vi "Close RF Subsystem Sessions.vi"(0 "RF SubSystem Session Providers":refnum<class "RF Subsystem Session Provider.lvclass">[](array[class]), 5 "TSM Context":T1, 11 "Error in":errorcluster) -> (15 "Error out":errorcluster)   [LabVIEW 2023, in "RFCalAndFixtureCharact.Common.lvlib"]
uses:
  RFCalAndFixtureCharact.Common.lvlib
  <vilib>/NI_TestStand_SemiconductorModule/NI_TestStand_Semiconductor_Module.lvlibp/PinMap/General/SemiconductorModuleContext.ctl
  RF Subsystem Session Provider/RF Subsystem Session Provider.lvclass
  <vilib>/NI_TestStand_SemiconductorModule/NI_TestStand_Semiconductor_Module.lvlibp
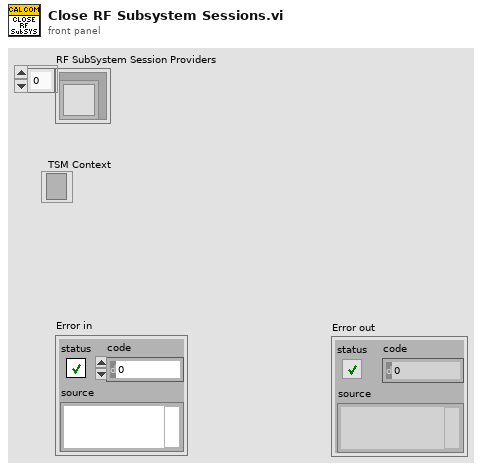
[diagram p1: front panel]
types:
  T1 = typedef "NI_TestStand_Semiconductor_Module.lvlibp/SemiconductorModuleContext.ctl" = refnum<k7>
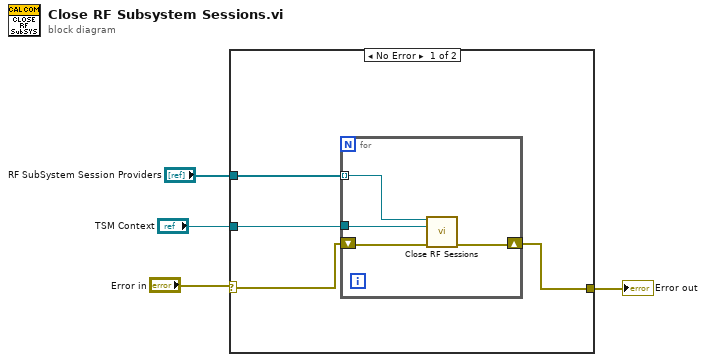
[diagram p0: block diagram]
diagram:
  n1 = case shown="No Error" "Error in" {
    selector: "Error in" -> [w6 w13]
    tunnel: [w8 w13] -> w4
    tunnel: "TSM Context" -> [w7 _]
    tunnel: "RF SubSystem Session Providers" -> [w5 _]
    frame No Error {
      n2 = for {
        shift-right: [w11] -> w8
        shift-left: w6 -> [w12]
        tunnel: w7 -> [w9]
        tunnel: w5 -> [w10] mode=indexing
        n3 = call-dynamic "Close RF Sessions.vi"("RF Subsystem Session Provider in"=w10, "TSM Context"=w9, "error in"=w12) -> ("error out"=w11:errorcluster)  [unwired: 11 in, 1 out]
      }
    }
    frame Error {
    }
  }
  "Error out" <- w4
